vi "Periodic Tasks.vi"(8 "error in":errorcluster) -> ()   [LabVIEW 2019]
doc: "This VI runs in parallel to other tasks. It can contain as many user-defined periodic loops as you need. These can carry out PID or other sorts of timed response."
uses:
  <vilib>/Rock Robotics/WPI/Utilities/WPI_GetSetVariantRefNum.vi
  <vilib>/Rock Robotics/Network Tables/NT Read Boolean.vi
  <vilib>/Rock Robotics/Network Tables/NT Read Number.vi
  <vilib>/addons/control/pid/pid.llb/PID (DBL).vi
  Robot Global Data.vi
  <vilib>/addons/control/pid/NI_PID_pid.lvlib
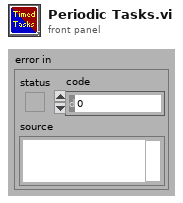
[diagram p1: front panel]
types:
  T1 = typedef "WPI_JoystickDevRef.ctl" = cluster{"Device":T2}
  T2 = typedef "WPI_JoystickDeviceEnum.ctl" = enum16{"USB 0", "USB 1", "USB 2", "USB 3", "USB 4", "USB 5"}
  T3 = cluster{"proportional gain (Kc)":dbl, "integral time (Ti, min)":dbl, "derivative time (Td, min)":dbl}
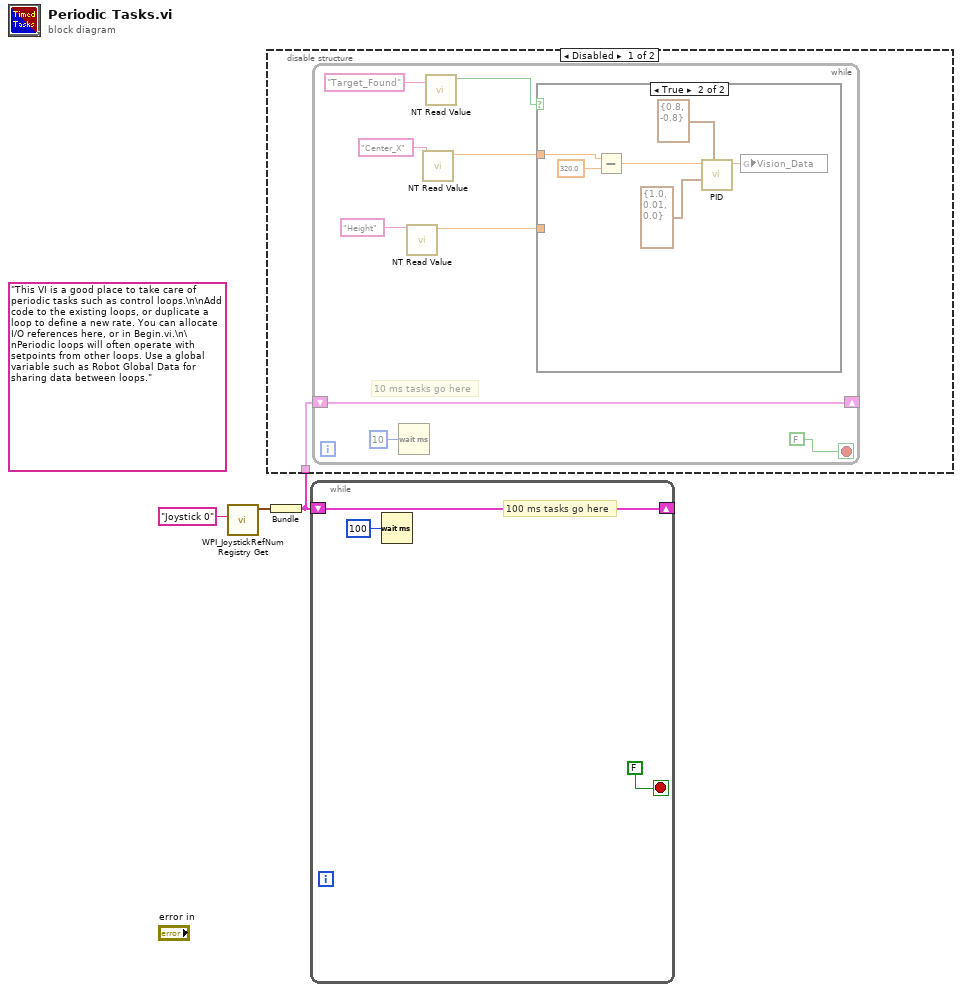
[diagram p0: block diagram]
diagram:
  (unwired) "This VI is a good place to take care of periodic tasks such as control loops.\n\nAdd code to the existing loops, or duplicate a loop to define a new rate. You can allocate I/O references here, or in Begin.vi.\n\nPeriodic loops will often operate with setpoints from other loops. Use a global variable such as Robot Global Data for sharing data between loops."
  n1 = call <vilib>:"WPI_JoystickRefNum Registry Get.vi"("refnum name"="Joystick 0") -> ("JoystickDevRef"=w2:T1)  [unwired: 1 in, 9 out]
  n2 = Bundle("JoystickDevRef"=w2) -> (w1:cluster{"JoystickDevRef":T1})  [unwired: 1 out]
  n3 = disable-structure shown="Disabled" {
    disable-tunnel: w1 -> [w4 _]
    frame Disabled {
      n4 = while {
        shift-right: [w11] -> _
        shift-left: w4 -> [w11]
        stop <- FALSE stop-if-true
        # "10 ms tasks go here"
        n5 = Wait (ms)(milliseconds to wait=u32 10) -> ()  [unwired: 1 out]
        n6 = call-poly <vilib>:"NT Read Value.vi"("Name"="Height") -> ("Numeric"=w5:dbl)  [unwired: 9 in, 1 out]
        n7 = call-poly <vilib>:"NT Read Value.vi"("Name"="Center_X") -> ("Numeric"=w6:dbl)  [unwired: 9 in, 1 out]
        n8 = call-poly <vilib>:"NT Read Value.vi"("Name"="Target_Found") -> ("Boolean"=w7:bool)  [unwired: 9 in, 1 out]
        n9 = case shown="True" w7 {
          tunnel: w6 -> [_ w19]
          tunnel: w5 -> [_ _]
          frame False {
          }
          frame True {
            n10 = Subtract(x=w19, y=320.0) -> (x-y=w17:dbl)
            n11 = call-poly <vilib>:"PID.vi"("output range"=cluster{"output high":dbl, "output low":dbl} {"output high"=0.8, "output low"=-0.8}, "PID gains"=T3 {"proportional gain (Kc)"=1.0, "integral time (Ti, min)"=0.01, "derivative time (Td, min)"=0.0}, "setpoint"=w17) -> ("output"=w14:dbl)  [unwired: 7 in, 1 out]
            n12 = global write "Robot Global Data.vi" "Vision_Data"(w14) -> ()
          }
        }
      }
    }
    frame Enabled {
    }
  }
  n13 = while {
    shift-right: [w20] -> _
    shift-left: w1 -> [w20]
    stop <- FALSE stop-if-true
    # "100 ms tasks go here"
    n14 = Wait (ms)(milliseconds to wait=u32 100) -> ()  [unwired: 1 out]
  }
